vi "Set_output_channel_group.vi"(8 "error in (no error)":errorcluster, 9 "Group_output":T1, 10 "Channel_output":dbl[](array[numeric]), 11 "Dali_usb_tridonics in":refnum<class "Dali_usb_tridonics.lvclass">) -> (0 "error out":errorcluster, 3 "Dali_usb_tridonics out":refnum<class "Dali_usb_tridonics.lvclass">)   [LabVIEW 2014, in "Driver_interaction.lvlib" / "Dali_usb_tridonics.lvclass"]
uses:
  Dali_usb_tridonics.lvclass
  Toolbox/Controls/Group_output.ctl
  Toolbox/Controls/Group_selector.ctl
  Dali_usb_tridonics.lvclass/Dali_usb_tridonics.ctl
  Vendor/Controls/Addressing_type.ctl
  _Driver_interaction/_Driver_interaction.lvclass
  Vendor/Dali_usb.lvlib
  Toolbox/Toolbox.lvclass
panel:
  out "Responses":string[](array[string])
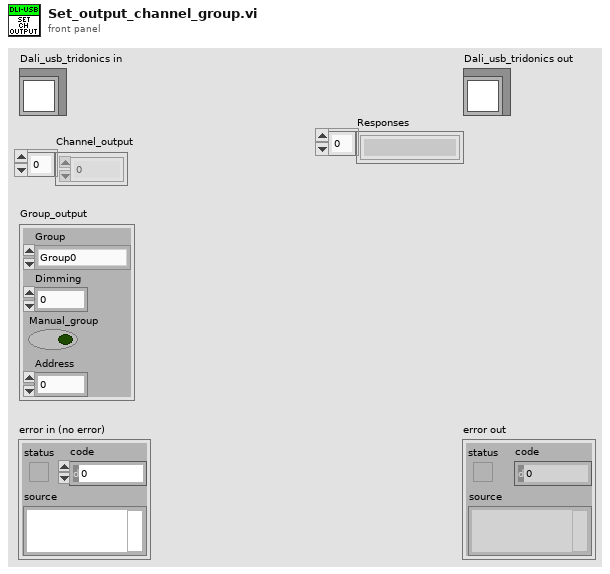
[diagram p1: front panel]
types:
  T1 = typedef "Driver_interaction.lvlib/Toolbox.lvclass/Group_output.ctl" = cluster{"Group":T2, "Dimming":i32, "Manual_group":bool, "Address":i32}
  T2 = typedef "Driver_interaction.lvlib/Toolbox.lvclass/Group_selector.ctl" = enum16{"Group0", "Group1", "Group2", "Group3", "Group4", "Group5", "Group6", "Group7", "Group8", "Group9", "Group10", "Group11", "Group12", "Group13", "Group14", "Group15", "All Groups"}
  T3 = typedef "Dali_usb.lvlib/Addressing_type.ctl" = string
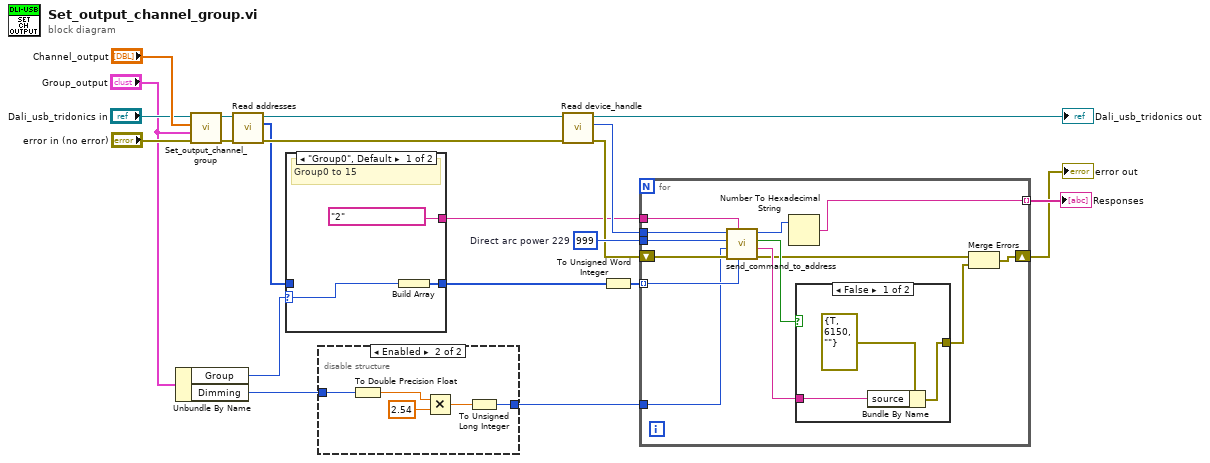
[diagram p0: block diagram]
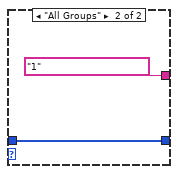
[diagram p2: hidden frame]
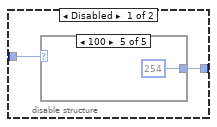
[diagram p3: hidden frame]
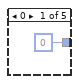
[diagram p4: hidden frame]
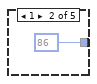
[diagram p5: hidden frame]
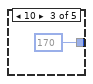
[diagram p6: hidden frame]
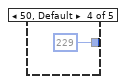
[diagram p7: hidden frame]
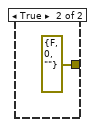
[diagram p8: hidden frame]
diagram:
  w16 = u32 999  # Direct arc power 229
  n1 = Unbundle By Name("Group_output") -> ("Group"=w4:T2, "Dimming"=w6:i32)
  n2 = call-parent "Set_output_channel_group.vi"("error in (no error)"="error in (no error)", "Group_output"="Group_output", "Channel_output"="Channel_output", "_Driver_interaction in"="Dali_usb_tridonics in") -> ("error out"=w11:errorcluster, "_Driver_interaction out"=w10:refnum<class "Dali_usb_tridonics.lvclass">)  [unwired: 6 in]
  n3 = call "Read addresses.vi"("error in (no error)"=w11, "Dali_usb_tridonics in"=w10) -> ("error out"=w17:errorcluster, "addresses"=w3:i32[], "Dali_usb_tridonics out"=w18:refnum<class "Dali_usb_tridonics.lvclass">)  [unwired: 7 in]
  n4 = case shown="\"Group0\", Default" w4 {
    selector: w4 -> [w22 _]
    tunnel: w3 -> [_ w26]
    tunnel: [w24 w26] -> w2
    tunnel: [T3 "2" ("addressing_type") T3 "1" ("addressing_type")] -> w1
    frame "Group0", Default {
      # "Group0 to 15"
      n5 = Build Array(w22) -> (w24:T2[])
    }
    frame "All Groups" {
    }
  }
  n6 = disable-structure shown="Enabled" {
    disable-tunnel: w6 -> [w28 w35]
    disable-tunnel: [w27 w34] -> w5
    frame Disabled {
      n7 = case shown="100" w28 {
        tunnel: [u32 0 ("unsigned 32bit integer") u32 86 ("unsigned 32bit integer") u32 170 ("unsigned 32bit integer") u32 229 ("unsigned 32bit integer") u32 254 ("unsigned 32bit integer")] -> w27
        frame 0 {
        }
        frame 1 {
        }
        frame 10 {
        }
        frame 50, Default {
        }
        frame 100 {
        }
      }
    }
    frame Enabled {
      n8 = To Double Precision Float(number=w35) -> (double precision float=w36:dbl)
      n9 = Multiply(x=w36, y=2.54) -> (x*y=w37:dbl)
      n10 = To Unsigned Long Integer(number=w37) -> (unsigned 32bit integer=w34:u32)
    }
  }
  n11 = call "Read device_handle.vi"("error in (no error)"=w17, "Dali_usb_tridonics in"=w18) -> ("error out"=w14:errorcluster, "device_handle"=w15:i32, "Dali_usb_tridonics out"=→"Dali_usb_tridonics out":refnum<class "Dali_usb_tridonics.lvclass">)  [unwired: 7 in]
  n12 = To Unsigned Word Integer(number=w2) -> (unsigned 16bit integer=w13:u16[])
  n13 = for {
    tunnel: w13 -> [w48] mode=indexing
    tunnel: w16 -> [w50]
    tunnel: w15 -> [w51]
    shift-right: [w41] -> w8
    shift-left: w14 -> [w49]
    tunnel: [w44] -> w12 mode=indexing
    tunnel: w5 -> [w40]
    tunnel: w1 -> [w39]
    n14 = call "send_command_to_address.vi"("address_group"=w48, "addressing_type"=w39, "error in (no error)"=w49, "command_data"=w40, "command"=w50, "device_handle"=w51) -> ("error out"=w43:errorcluster, "failstring"=w46:string, "ok"=w47:bool, "response_command"=w45:i32)  [unwired: 2 in]
    n15 = Number To Hexadecimal String(2:w45) -> (0:w44:string)  [unwired: 1 in]
    n16 = case shown="False" w47 {
      tunnel: w46 -> [w53 _]
      tunnel: [w52 errorcluster {"status"=FALSE, "code"=0, "source"=""} ("error out")] -> w42
      frame False {
        n17 = Bundle By Name(cluster=errorcluster {"status"=TRUE, "code"=6150, "source"=""} ("error out"), "source"=w53) -> (w52:errorcluster)
      }
      frame True {
      }
    }
    n18 = Merge Errors(w43, w42) -> (w41:errorcluster)
  }
  "error out" <- w8
  "Responses" <- w12
